vi "Depositos de agua comunicados.vi"() -> ()   [LabVIEW 2018]
panel:
  out "Electrovalcula":bool
  out "Tanque B":dbl(slide) scale=0.0..3.65
  out "Tanque A":dbl(slide) scale=0.0..3.65
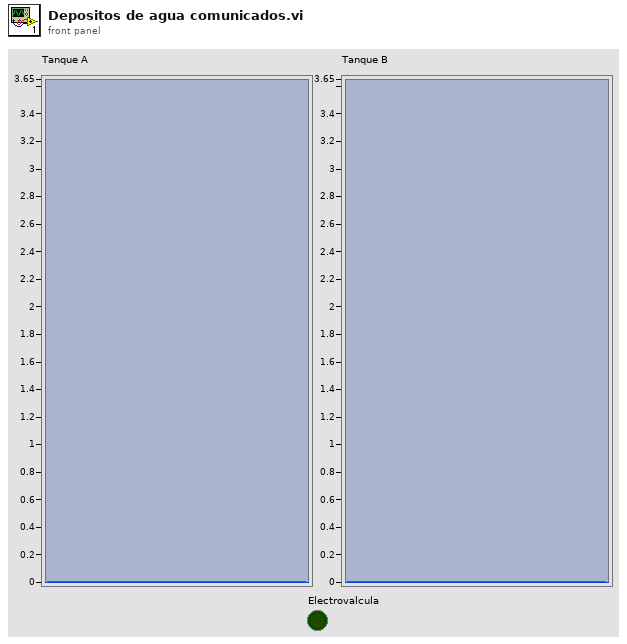
[diagram p1: front panel]
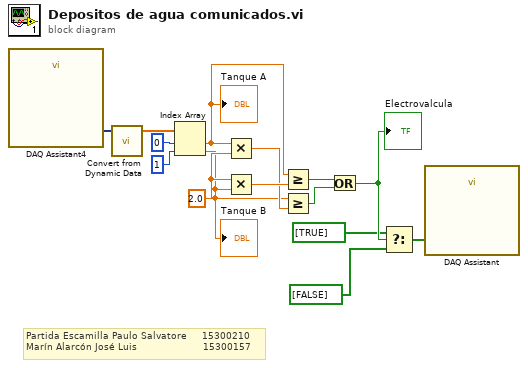
[diagram p0: block diagram]
diagram:
  w11 = 2.0 ("x")
  # "Partida Escamilla Paulo Salvatore     15300210\nMarín Alarcón José Luis                      15300157"
  n1 = call "DAQ Assistant4"() -> ("data"=w15:dynamicdata)  [unwired: 17 in, 2 out]
  n2 = call "Convert from Dynamic Data"("Dynamic Data Type"=w15) -> ("Array"=w14:dbl[])  [unwired: 3 in]
  n3 = Index Array(array=w14, index #1=0 ("index"), index #2=1 ("index")) -> (element #1=w4:dbl, element #2=w5:dbl)
  "Tanque A" <- w4
  "Tanque B" <- w5
  n4 = Multiply(x=w4, y=w11) -> (x*y=w9:dbl)
  n5 = Multiply(x=w11, y=w5) -> (x*y=w10:dbl)
  n6 = Greater Or Equal?(x=w4, y=w10) -> (x >= y?=w8:bool)
  n7 = Greater Or Equal?(x=w5, y=w9) -> (x >= y?=w7:bool)
  n8 = Or(x=w8, y=w7) -> (x .or. y?=w6:bool)
  "Electrovalcula" <- w6
  n9 = Select(t=bool[] [TRUE] ("data"), s=w6, f=bool[] [FALSE] ("data")) -> (s? t:f=w1:bool[])
  n10 = call "DAQ Assistant"("data"=w1) -> ()  [unwired: 17 in, 2 out]
